vi "ReadWFGSettings.vi"(0 "object in":refnum<class "AD2andExtAWG.lvclass">, 5 "error in (no error)":errorcluster) -> (14 "object out":refnum<class "AD2andExtAWG.lvclass">, 16 "AmplitudeAndVoltage":T1, 19 "error out":errorcluster)   [LabVIEW 2019, in "AD2andExtAWG.lvclass"]
uses:
  AD2andExtAWG.lvclass
  AFG3022B_class/AFG3022B.lvclass
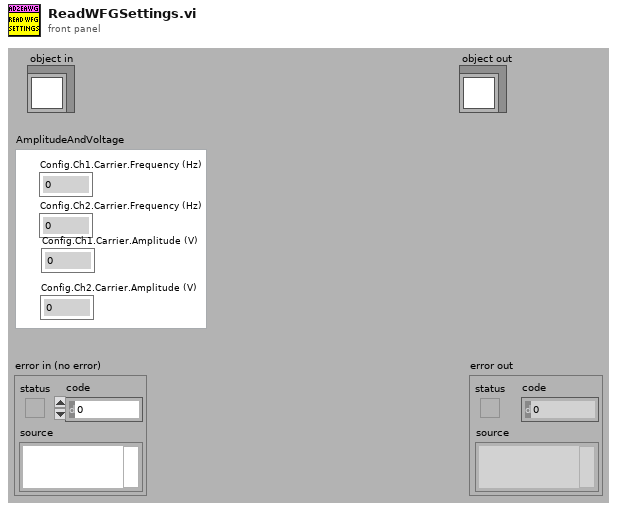
[diagram p1: front panel]
types:
  T1 = cluster{"Config.Ch1.Carrier.Frequency (Hz)":dbl, "Config.Ch2.Carrier.Frequency (Hz)":dbl, "Config.Ch1.Carrier.Amplitude (V)":dbl, "Config.Ch2.Carrier.Amplitude (V)":dbl}
  T2 = cluster{"ConfigDataCh1":cluster{"Frequency Hz (1000 Hz)":dbl, "Waveform Function (0: Sine)":u16, "Amplitude (1 Vpp)":dbl, "DC Offset (0.00 V)":dbl, "Phase Level (-1)":dbl, "Phase Unit (0: Radian)":u16}, "ConfigDataCh2":cluster{"Frequency Hz (1000 Hz)":dbl, "Waveform Function (0: Sine)":u16, "Amplitude (1 Vpp)":dbl, "DC Offset (0.00 V)":dbl, "Phase Level (-1)":dbl, "Phase Unit (0: Radian)":u16}}
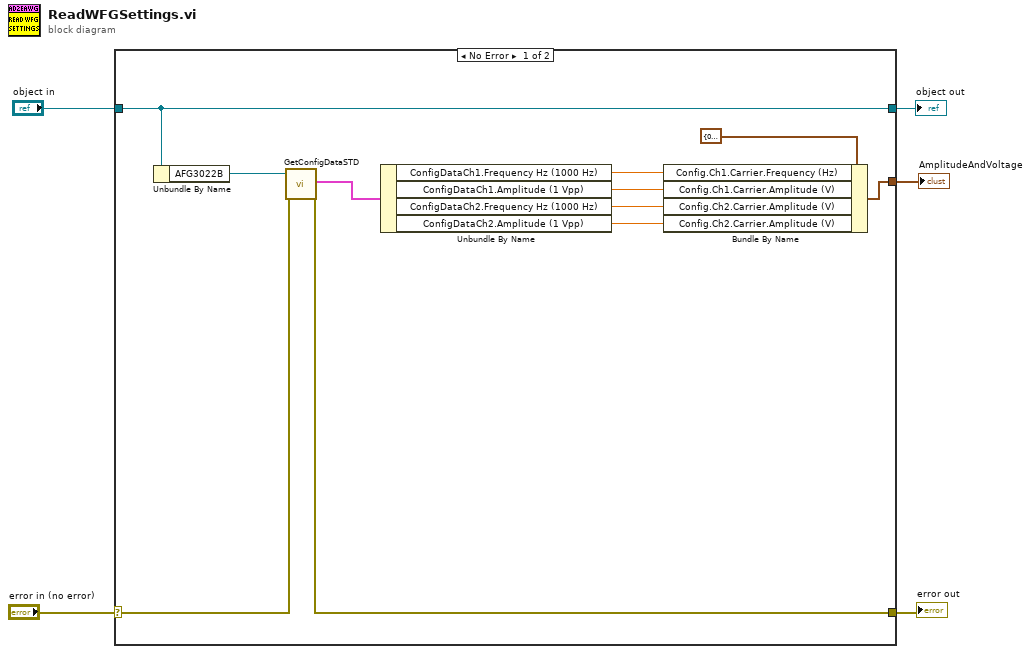
[diagram p0: block diagram]
diagram:
  n1 = case shown="No Error" "error in (no error)" {
    selector: "error in (no error)" -> [w10 w18]
    tunnel: [w9 w18] -> w4
    tunnel: [w16 w17] -> w2
    tunnel: "object in" -> [w16 w17]
    tunnel: [w8 _] -> w1
    frame No Error {
      n2 = Unbundle By Name(w16) -> ("AFG3022B"=w15:refnum<class "AFG3022B.lvclass">)
      n3 = call-dynamic "GetConfigDataSTD.vi"("object in"=w15, "error in (no error)"=w10) -> ("Configdatastd"=w11:T2, "error out"=w9:errorcluster)  [unwired: 15 in, 1 out]
      n4 = Unbundle By Name(w11) -> ("ConfigDataCh1.Frequency Hz (1000 Hz)"=w13:dbl, "ConfigDataCh1.Amplitude (1 Vpp)"=w12:dbl, "ConfigDataCh2.Frequency Hz (1000 Hz)"=w7:dbl, "ConfigDataCh2.Amplitude (1 Vpp)"=w6:dbl)
      n5 = Bundle By Name(cluster=T1 {"Config.Ch1.Carrier.Frequency (Hz)"=0.0, "Config.Ch2.Carrier.Frequency (Hz)"=0.0, "Config.Ch1.Carrier.Amplitude (V)"=0.0, "Config.Ch2.Carrier.Amplitude (V)"=0.0} ("AmplitudeAndVoltage"), "Config.Ch1.Carrier.Frequency (Hz)"=w13, "Config.Ch1.Carrier.Amplitude (V)"=w12, "Config.Ch2.Carrier.Amplitude (V)"=w7, "Config.Ch2.Carrier.Amplitude (V)"=w6) -> (w8:T1)
    }
    frame Error {
    }
  }
  "error out" <- w4
  "object out" <- w2
  "AmplitudeAndVoltage" <- w1
